vi "Write Digital Channel.vi"   [LabVIEW 2020, in "BDAQ-6104.lvlib"]
uses:
  <instrlib>/BDAQ-6104/BDAQ-6104.lvlib
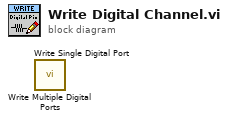
[diagram p0: block diagram]
diagram:
  n1 = call <instrlib>:"Write Multiple Digital Ports.vi"() -> ()  [unwired: 10 in, 2 out]
  n2 = call <instrlib>:"Write Single Digital Port.vi"() -> ()  [unwired: 10 in, 2 out]
